vi "Read GameRef.vi"(8 "error in (no error)":errorcluster, 11 "PassObjective in":refnum<class "PassObjective.lvclass">) -> (0 "error out":errorcluster, 2 "GameRef":refnum<data-value>, 3 "PassObjective out":refnum<class "PassObjective.lvclass">)   [LabVIEW 2023, in "PassObjective.lvclass"]
uses:
  PassObjective.lvclass
  Game_class/Game.lvclass
  PassObjective.lvclass/PassObjective.ctl
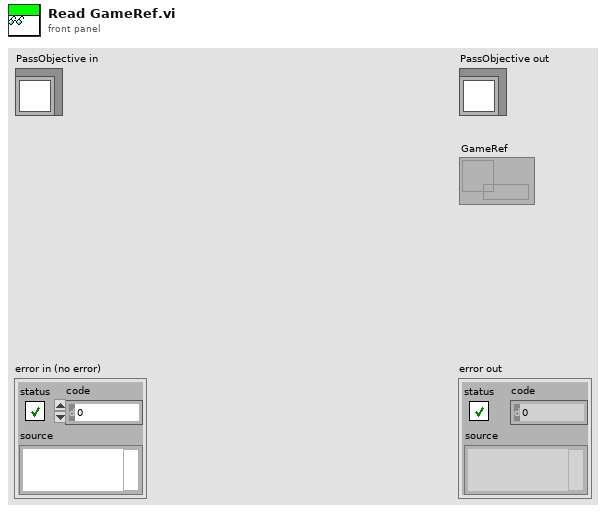
[diagram p1: front panel]
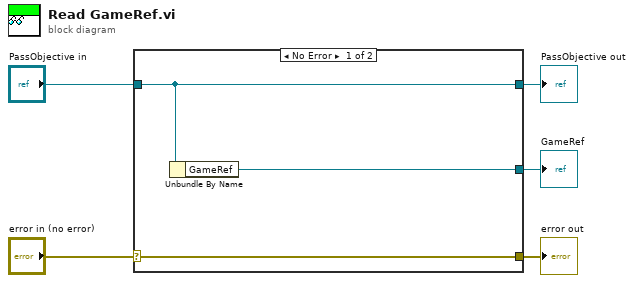
[diagram p0: block diagram]
diagram:
  n1 = case shown="No Error" "error in (no error)" {
    selector: "error in (no error)" -> [w8 w9]
    tunnel: [w8 w9] -> w4
    tunnel: [w7 w10] -> w2
    tunnel: "PassObjective in" -> [w7 w10]
    tunnel: [w6 _] -> w1
    frame No Error {
      n2 = Unbundle By Name(w7) -> ("GameRef"=w6:refnum<data-value>)
    }
    frame Error {
    }
  }
  "error out" <- w4
  "PassObjective out" <- w2
  "GameRef" <- w1
